vi "Configure Reporting Dialog.vi"(8 "error in (no error)":errorcluster, 11 "Execution UI In":refnum<class "Execution UI.lvclass">) -> (0 "error out":errorcluster, 2 "Reporting Enabled?":bool, 3 "Execution UI Out":refnum<class "Execution UI.lvclass">)   [LabVIEW 2020, in "Execution UI.lvclass"]
uses:
  Execution UI.lvclass
  Framework/Report Interface/Report Interface.lvclass
  Framework/Report/Report.lvclass
  <vilib>/Utility/sysdir.llb/Get System Directory.vi
  <vilib>/Utility/libraryn.llb/Create Directory Recursive.vi
  Configuration Manager/Configuration Manager.lvclass
  Support/Paths.lvlib
  Plugin Loader/Plugin Loader.lvclass
  Framework/Plugin/Plugin.lvclass
panel:
  in  "Reports Plugins":i32(listbox)
  in  "Configure":bool
  in  "Commit":bool
  in  "Cancel":bool
  # "Double Click to toggle active plugin"
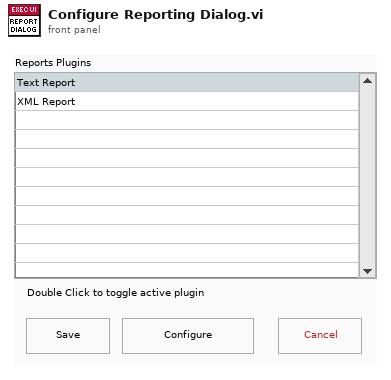
[diagram p1: front panel]
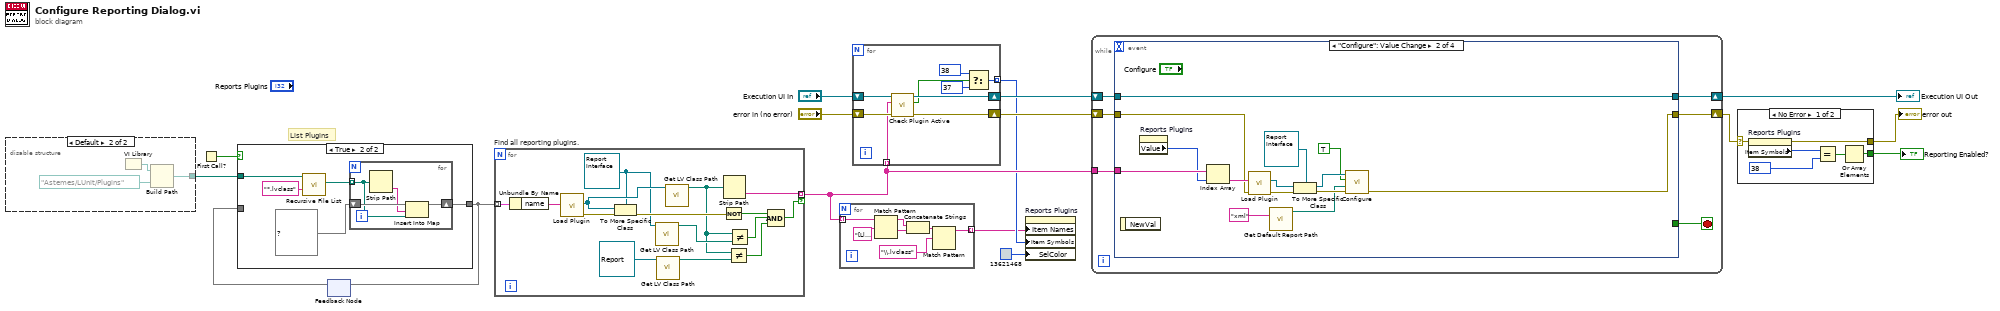
[diagram p0: block diagram]
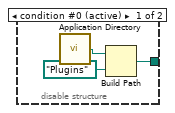
[diagram p2: hidden frame]
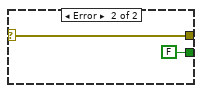
[diagram p4: hidden frame]
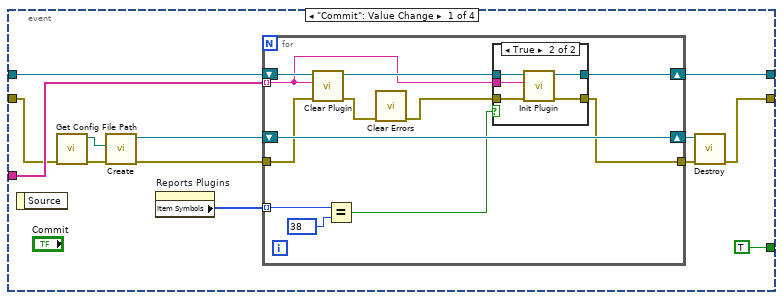
[diagram p5: hidden frame]
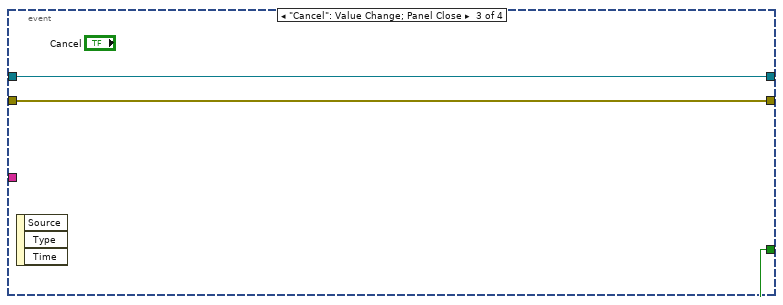
[diagram p7: hidden frame]
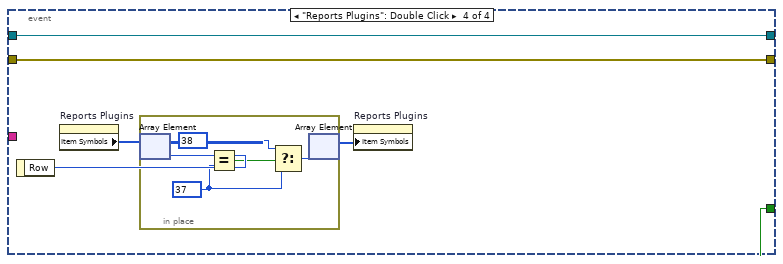
[diagram p8: hidden frame]
diagram:
  # "List Plugins"
  n1 = disable-structure shown="Default" {
    disable-tunnel: [w17 w20] -> w5
    frame condition #0 (active) {
      n2 = call <vilib>:"Application Directory.vi"() -> ("Application Directory"=w19:path)
      n3 = Build Path(base path=w19, name or relative path=path "Plugins") -> (appended path=w17:path)
    }
    frame condition #1 {
      n4 = VI Library() -> (path=w22:path)
      n5 = Build Path(base path=w22, name or relative path=path "Astemes/LUnit/Plugins") -> (appended path=w20:path)
    }
  }
  n6 = First Call?() -> (First Call?: T/F=w8:bool)
  n7 = feedback #1() -> (w9:map{string, path})  [unwired: 1 in]
  n8 = case shown="True" w8 {
    tunnel: w5 -> [_ w25]
    tunnel: [w23 w24] -> w10
    tunnel: w9 -> [w23 _]
    frame False {
    }
    frame True {
      n9 = call <vilib>:"Recursive File List.vi"("pattern"="*.lvclass", "Folder Path"=w25) -> ("All Files in Dir"=w26:path[])  [unwired: 5 in, 4 out]
      n10 = for {
        shift-right: [w31] -> w24
        shift-left: map{string, path} {} ("map") -> [w32]
        tunnel: w26 -> [w29] mode=indexing
        n11 = Strip Path(path=w29) -> (name=w30:string)  [unwired: 1 out]
        n12 = Insert Into Map(map in=w32, key=w30, value=w29) -> (map out=w31:map{string, path})  [unwired: 2 out]
      }
    }
  }
  n13 = feedback-in #1(w10) -> ()
  n14 = for "Find all reporting plugins." {
    tunnel: w10 -> [w47] mode=indexing
    tunnel: [w42] -> w11 mode=indexing if=w41
    w38 = refnum<class "Report Interface.lvclass"> refnum ("Reports.lvlib:Report Interface.lvclass")
    n15 = Unbundle By Name(w47) -> ("name"=w33:string)
    n16 = call "Load Plugin.vi"("Plugin"=w33) -> ("error out"=w46:errorcluster, "Plugin"=w45:refnum<class "Plugin.lvclass">)  [unwired: 9 in]
    n17 = To More Specific Class(target class=w38, reference=w45, error in=w46) -> (error out=w44:errorcluster)  [unwired: 1 out]
    n18 = call <vilib>:"Get LV Class Path.vi"("object"=w38) -> ("class path"=w40:path)  [unwired: 9 in, 1 out]
    n19 = call <vilib>:"Get LV Class Path.vi"("object"=refnum<class "Report.lvclass"> refnum ("Reports.lvlib:Report.lvclass")) -> ("class path"=w36:path)  [unwired: 9 in, 1 out]
    n20 = call <vilib>:"Get LV Class Path.vi"("object"=w45) -> ("class path"=w35:path)  [unwired: 9 in, 1 out]
    n21 = Not(x=w44) -> (.not. x?=w43:bool)
    n22 = Strip Path(path=w35) -> (name=w42:string)  [unwired: 1 out]
    n23 = Not Equal?(x=w35, y=w36) -> (x != y?=w34:bool)
    n24 = Not Equal?(x=w35, y=w40) -> (x != y?=w39:bool)
    n25 = Compound Arithmetic op=AND(w43, w39, w34) -> (w41:bool)
  }
  n26 = for {
    tunnel: w11 -> [w53] mode=indexing
    tunnel: [w50] -> w6 mode=indexing
    n27 = Match Pattern(string=w53, regular expression="[Ll][Uu][Nn][Ii][Tt] ") -> (before substring=w48:string, after substring=w52:string)  [unwired: 1 in, 2 out]
    n28 = Concatenate Strings(w48, w52) -> (w49:string)
    n29 = Match Pattern(string=w49, regular expression="\\.lvclass") -> (before substring=w50:string)  [unwired: 1 in, 3 out]
  }
  n30 = for {
    shift-right: [w62] -> w14
    shift-left: "Execution UI In" -> [w63]
    shift-right: [w60] -> w12
    shift-left: "error in (no error)" -> [w61]
    tunnel: w11 -> [w59] mode=indexing
    tunnel: [w55] -> w7 mode=indexing
    n31 = call "Check Plugin Active.vi"("error in (no error)"=w61, "Plugin"=w59, "Execution UI in"=w63) -> ("error out"=w60:errorcluster, "Active?"=w56:bool, "Execution UI out"=w62:refnum<class "Execution UI.lvclass">)  [unwired: 6 in]
    n32 = Select(t=38, s=w56, f=37) -> (s? t:f=w55:i32)
  }
  n33 = property on="Reports Plugins" class="LstBox (strict)"("Item Names"=w6, "Item Symbols"=w7, "SelColor"=u32 13621468 ("Primary Light")) -> ()  [unwired: 2 in, 2 out]
  n34 = while {
    tunnel: w11 -> [w65]
    shift-right: [w69] -> w16
    shift-left: w14 -> [w67]
    shift-right: [w68] -> w3
    shift-left: w12 -> [w66]
    stop <- w64 stop-if-true
    n35 = event shown="[1] \"Configure\": Value Change" {
      selector: _ -> [_ _ _ _]
      dyn-events: _ -> [_ _ _ _]
      timeout: _ -> [_ _ _ _]
      tunnel: [w80 w105 w117 w121] -> w69
      tunnel: w67 -> [w82 w105 w117 w121]
      tunnel: w66 -> [w70 w104 w118 w120]
      tunnel: [w81 w107 w118 w120] -> w68
      tunnel: w65 -> [w79 w115 _ _]
      tunnel: [TRUE _ TRUE FALSE] -> w64
      event "Commit": Value Change {
        n36 = event-data() -> ()  [unwired: 1 in, 1 out]
        n37 = call "Get Config File Path.vi"("error in (no error)"=w70) -> ("error out"=w76:errorcluster, "Config Directory"=w75:path)  [unwired: 9 in]
        n38 = call "Create.vi"("error in (no error)"=w76, "configuration file path"=w75) -> ("error out"=w71:errorcluster, "Configuration Manager out"=w77:refnum<class "Configuration Manager.lvclass">)  [unwired: 8 in]
        n39 = property on="Reports Plugins" class="LstBox (strict)"() -> ("Item Symbols"=w72:i32[])  [unwired: 2 in, 2 out]
        n40 = for {
          tunnel: w79 -> [w85] mode=indexing
          tunnel: [w86] -> w74
          shift-right: [w91] -> w80
          shift-left: w82 -> [w94]
          shift-right: [w89] -> w73
          shift-left: w77 -> [w89]
          tunnel: w72 -> [w88] mode=indexing
          tunnel: w71 -> [w83]
          n41 = call "Clear Plugin.vi"("error in (no error)"=w83, "Plugin"=w85, "Execution UI in"=w94) -> ("error out"=w90:errorcluster, "Execution UI out"=w92:refnum<class "Execution UI.lvclass">)  [unwired: 7 in]
          n42 = Equal?(x=w88, y=38) -> (x = y?=w84:bool)
          n43 = call <vilib>:"Clear Errors.vi"("error in (no error)"=w90) -> ("error out"=w93:errorcluster)  [unwired: 5 in, 1 out]
          n44 = case shown="True" w84 {
            tunnel: w93 -> [w96 w101]
            tunnel: w92 -> [w95 w100]
            tunnel: [w95 w99] -> w91
            tunnel: [w96 w98] -> w86
            tunnel: w85 -> [_ w97]
            frame False {
            }
            frame True {
              n45 = call "Init Plugin.vi"("error in (no error)"=w101, "Plugin"=w97, "Execution UI in"=w100) -> ("error out"=w98:errorcluster, "Execution UI out"=w99:refnum<class "Execution UI.lvclass">)  [unwired: 7 in]
            }
          }
        }
        n46 = call "Destroy.vi"("error in (no error)"=w74, "Configuration Manager In"=w73) -> ("error out"=w81:errorcluster)  [unwired: 9 in]
      }
      event "Configure": Value Change {
        n47 = event-data() -> ()  [unwired: 1 in, 1 out]
        n48 = property on="Reports Plugins" class="LstBox (strict)"() -> ("Value"=w114:i32)  [unwired: 2 in, 2 out]
        n49 = Index Array(array=w115, index=w114) -> (element=w113:string)
        n50 = call "Load Plugin.vi"("error in (no error)"=w104, "Plugin"=w113) -> ("error out"=w110:errorcluster, "Plugin"=w111:refnum<class "Plugin.lvclass">)  [unwired: 8 in]
        n51 = call "Get Default Report Path.vi"("File Extension"="xml") -> ("Default Report Path"=w102:path)  [unwired: 9 in, 1 out]
        n52 = To More Specific Class(target class=refnum<class "Report Interface.lvclass"> refnum ("Reports.lvlib:Report Interface.lvclass"), reference=w111, error in=w110) -> (specific class reference=w109:refnum<class "Report Interface.lvclass">, error out=w108:errorcluster)
        n53 = call-dynamic "Configure.vi"("error in (no error)"=w108, "Default Path"=w102, "Interactive?"=TRUE, "Report Interface in"=w109) -> ("error out"=w107:errorcluster)  [unwired: 6 in, 1 out]
      }
      event "Cancel": Value Change; Panel Close {
        n54 = event-data() -> ()  [unwired: 1 in, 3 out]
      }
      event "Reports Plugins": Double Click {
        n55 = event-data() -> ("Row"=w123:i32)  [unwired: 1 in]
        n56 = property on="Reports Plugins" class="LstBox (strict)"() -> ("Item Symbols"=w124:i32[])  [unwired: 2 in, 2 out]
        n57 = in-place {
          w127 = 37
          n58 = in-place-array #2(w124, w123) -> (w129:i32)
          n59 = Equal?(x=w129, y=w127) -> (x = y?=w126:bool)
          n60 = Select(t=38, s=w126, f=w127) -> (s? t:f=w125:i32)
          n61 = in-place-array #2(w125) -> (w122:i32[])  [unwired: 1 out]
        }
        n62 = property on="Reports Plugins" class="LstBox (strict)"("Item Symbols"=w122) -> ()  [unwired: 2 in, 2 out]
      }
    }
  }
  "Execution UI Out" <- w16
  n63 = case shown="No Error" w3 {
    selector: w3 -> [w131 w137]
    tunnel: [w132 FALSE] -> w2
    tunnel: [w130 w137] -> w1
    frame No Error {
      n64 = property on="Reports Plugins" class="LstBox (strict)"(error in=w131) -> (error out=w130:errorcluster, "Item Symbols"=w135:i32[])  [unwired: 1 in, 1 out]
      n65 = Equal?(x=w135, y=38) -> (x = y?=w133:bool[])
      n66 = Or Array Elements(Boolean array=w133) -> (logical OR=w132:bool)
    }
    frame Error {
    }
  }
  "error out" <- w1
  "Reporting Enabled?" <- w2
